vi "Joystick 2 Manual Control.vi"(11 "Buttons":T1) -> (0 "Shooter Motor Out":dbl=0.1, 1 "Roller Motor Out":dbl, 2 "Arm Out":T3, 3 "Compressor Relay Out":T2)   [LabVIEW 2013]
uses:
  <vilib>/Rock Robotics/WPI/Solenoid/WPI_SolenoidValue.ctl
  <vilib>/Rock Robotics/WPI/Relay/WPI_RelayValue.ctl
  Joystick 2.ctl
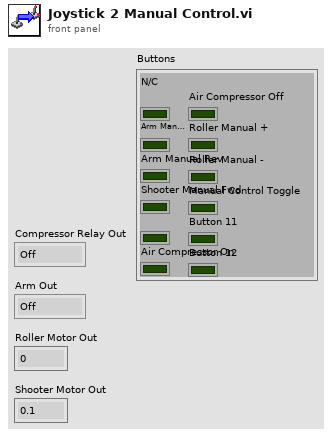
[diagram p1: front panel]
types:
  T1 = typedef "Joystick 2.ctl" = cluster{"N/C":bool, "Arm Manual Fwd":bool, "Arm Manual Rev":bool, "Shooter Manual Fwd":bool, bool, "Air Compressor On":bool, "Air Compressor Off":bool, "Roller Manual +":bool, "Roller Manual -":bool, "Manual Control Toggle":bool, "Button 11":bool, "Button 12":bool}
  T2 = typedef "WPI_RelayValue.ctl" = enum16{"Off", "On", "Forward", "Reverse"}
  T3 = typedef "WPI_SolenoidValue.ctl" = enum16{"Off", "On", "Forward", "Reverse"}
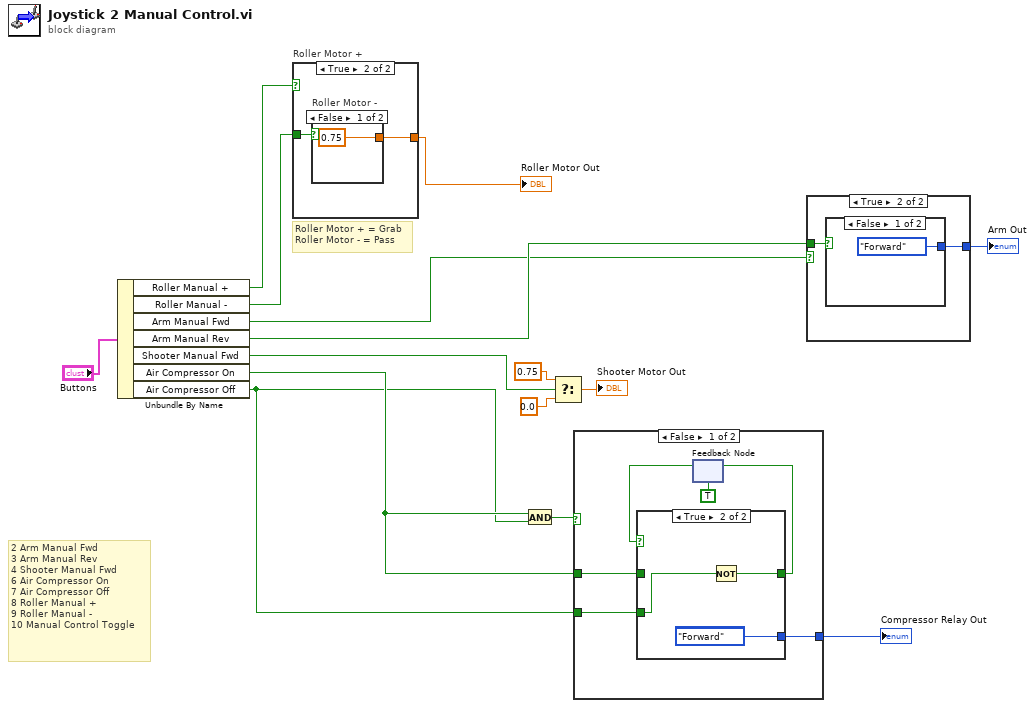
[diagram p0: block diagram]
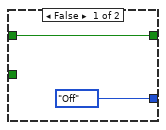
[diagram p2: hidden frame]
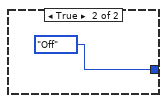
[diagram p3: hidden frame]
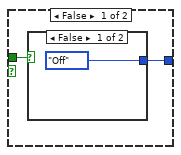
[diagram p4: hidden frame]
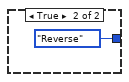
[diagram p5: hidden frame]
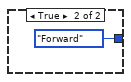
[diagram p6: hidden frame]
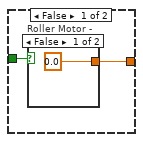
[diagram p7: hidden frame]
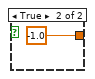
[diagram p8: hidden frame]
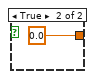
[diagram p9: hidden frame]
diagram:
  # "Roller Motor + = Grab\nRoller Motor - = Pass"
  # "2 Arm Manual Fwd\n3 Arm Manual Rev\n4 Shooter Manual Fwd\n6 Air Compressor On\n7 Air Compressor Off\n8 Roller Manual +\n9 Roller Manual -\n10 Manual Control Toggle"
  n1 = Unbundle By Name("Buttons") -> ("Roller Manual +"=w10:bool, "Roller Manual -"=w9:bool, "Arm Manual Fwd"=w5:bool, "Arm Manual Rev"=w7:bool, "Shooter Manual Fwd"=w12:bool, "Air Compressor On"=w2:bool, "Air Compressor Off"=w1:bool)
  n2 = case "Roller Motor +" shown="True" w10 {
    tunnel: w9 -> [w17 w21]
    tunnel: [w16 w20] -> w8
    frame False {
      n3 = case "Roller Motor -" shown="False" w17 {
        tunnel: [0.0 -1.0] -> w16
        frame False {
        }
        frame True {
        }
      }
    }
    frame True {
      n4 = case "Roller Motor -" shown="False" w21 {
        tunnel: [0.75 ("t") 0.0 ("t")] -> w20
        frame False {
        }
        frame True {
        }
      }
    }
  }
  "Roller Motor Out" <- w8
  n5 = And(x=w2, y=w1) -> (x .and. y?=w4:bool)
  n6 = Select(t=0.75, s=w12, f=0.0) -> (s? t:f=→"Shooter Motor Out":dbl)
  n7 = case shown="False" w4 {
    tunnel: w2 -> [w26 _]
    tunnel: w1 -> [w25 _]
    tunnel: [w24 WPI_RelayValue."Off" ("RelayValue")] -> w3
    frame False {
      n8 = feedback #1(TRUE ("Air Compressor On")) -> (w28:bool)
      n9 = case shown="True" w28 {
        tunnel: w26 -> [w30 _]
        tunnel: [w30 w32] -> w29
        tunnel: [WPI_RelayValue."Off" ("RelayValue") WPI_RelayValue."Forward" ("RelayValue")] -> w24
        tunnel: w25 -> [_ w33]
        frame False {
        }
        frame True {
          (unwired) WPI_RelayValue."Forward" ("RelayValue")
          n10 = Not(x=w33) -> (.not. x?=w32:bool)
        }
      }
      n11 = feedback-in #1(w29) -> ()
    }
    frame True {
    }
  }
  "Compressor Relay Out" <- w3
  n12 = case shown="True" w5 {
    tunnel: [w37 w41] -> w6
    tunnel: w7 -> [w36 w40]
    frame False {
      n13 = case shown="False" w36 {
        tunnel: [WPI_SolenoidValue."Off" ("Value") WPI_SolenoidValue."Reverse" ("Value")] -> w37
        frame False {
        }
        frame True {
        }
      }
    }
    frame True {
      n14 = case shown="False" w40 {
        tunnel: [WPI_SolenoidValue."Forward" ("Value") WPI_SolenoidValue."Forward" ("Value")] -> w41
        frame False {
        }
        frame True {
        }
      }
    }
  }
  "Arm Out" <- w6
